vi "Stufen gleichmäßig aufteilen.vi"(8 "Punkte umkehren":bool, 10 "Stufen":u16, 11 "Anzahl":u16) -> (3 "Stufen":u16[](array[numeric]))   [LabVIEW 2020, in "Linearisierung v2.lvlib" / "Gasteiler.lvlib"]
uses:
  Gasteiler.lvlib
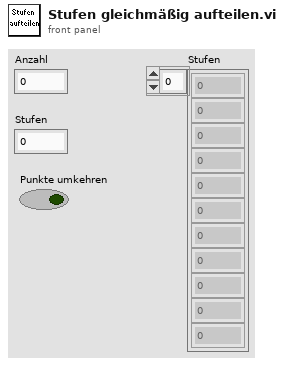
[diagram p1: front panel]
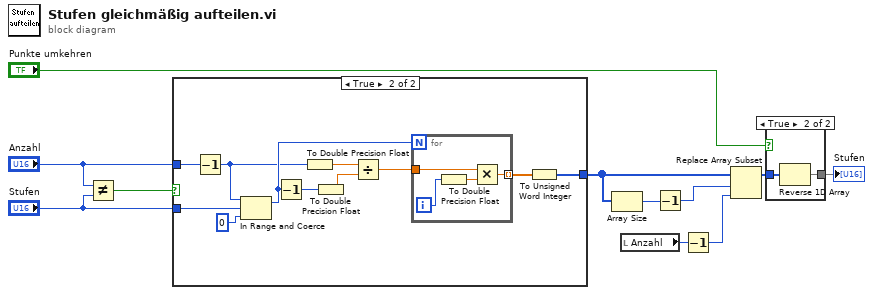
[diagram p0: block diagram]
diagram:
  n1 = Not Equal?(x="Anzahl", y="Stufen") -> (x != y?=w2:bool)
  n2 = case shown="True" w2 {
    tunnel: "Stufen" -> [_ w25]
    tunnel: "Anzahl" -> [w12 w22]
    tunnel: [w13 w19] -> w7
    frame False {
      n3 = for {
        N: w12 -> [_]
        tunnel: [w14] -> w13 mode=indexing
        i -> [w14]
      }
    }
    frame True {
      n4 = Decrement(x=w22) -> (x-1=w21:u16)
      n5 = In Range and Coerce(upper limit=w21, x=w25, lower limit=u16 0 ("Untergrenze")) -> (coerced(x)=w24:u16)  [unwired: 1 out]
      n6 = Decrement(x=w24) -> (x-1=w15:u16)
      n7 = To Double Precision Float(number=w21) -> (double precision float=w17:dbl)
      n8 = To Double Precision Float(number=w15) -> (double precision float=w16:dbl)
      n9 = Divide(x=w17, y=w16) -> (x/y=w18:dbl)
      n10 = for {
        N: w24 -> [_]
        tunnel: w18 -> [w29]
        tunnel: [w28] -> w20 mode=indexing
        i -> [w26]
        n11 = To Double Precision Float(number=w26) -> (double precision float=w27:dbl)
        n12 = Multiply(x=w29, y=w27) -> (x*y=w28:dbl)
      }
      n13 = To Unsigned Word Integer(number=w20) -> (unsigned 16bit integer=w19:u16[])
    }
  }
  n14 = Array Size(array=w7) -> (size(s)=w11:i32)
  n15 = local read "Anzahl"() -> (w9:u16)
  n16 = Decrement(x=w11) -> (x-1=w10:i32)
  n17 = Decrement(x=w9) -> (x-1=w8:u16)
  n18 = Replace Array Subset(array=w7, new element=w8, index=w10) -> (w6:i32[])
  n19 = case shown="True" "Punkte umkehren" {
    tunnel: w6 -> [w30 w32]
    tunnel: [w30 w31] -> w5
    frame False {
    }
    frame True {
      n20 = Reverse 1D Array(array=w32) -> (reversed array=w31:i32[])
    }
  }
  "Stufen" <- w5
